vi "Detect and Decode Multiple.vi"   [LabVIEW 2020, in "feature_detection.lvlib" / "QR Code Detector.lvclass"]
doc: "Perform the Detection and Decoding steps on an Image which can contain multiple QR Codes."
uses:
  QR Code Detector.lvclass
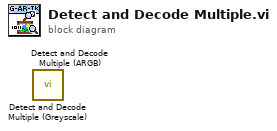
[diagram p0: block diagram]
diagram:
  n1 = call "Detect and Decode Multiple (Greyscale).vi"() -> ()  [unwired: 9 in, 3 out]
  n2 = call "Detect and Decode Multiple (ARGB).vi"() -> ()  [unwired: 9 in, 3 out]
